vi "Config Data to String.vi"(1 "data":T1[](array[typedef]), 2 "section names":string[](array[string])) -> (0 "string":string)   [LabVIEW 2009]
uses:
  Config Data Section.ctl
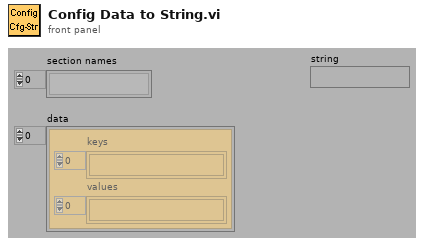
[diagram p1: front panel]
types:
  T1 = typedef "Config Data Section.ctl" = cluster{"keys":string[], "values":string[]}
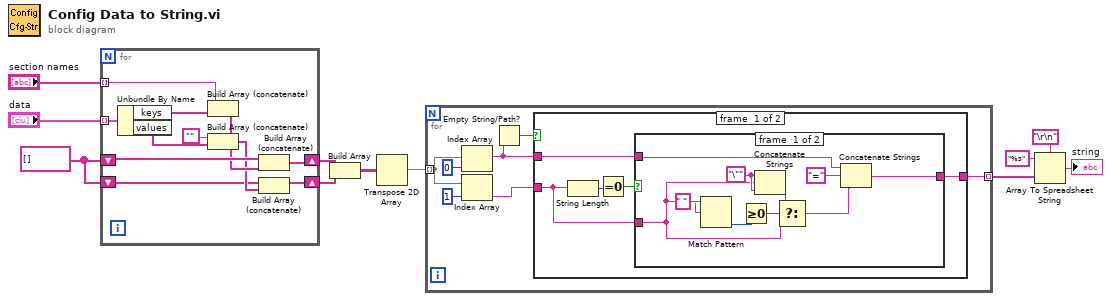
[diagram p0: block diagram]
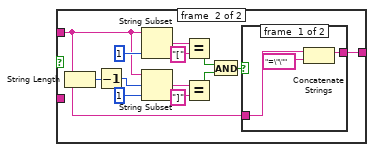
[diagram p2: hidden frame]
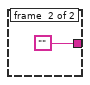
[diagram p4: hidden frame]
diagram:
  w3 = string[] []
  n1 = for {
    tunnel: "data" -> [w22] mode=indexing
    shift-right: [w18] -> w4
    shift-left: w3 -> [w17]
    shift-right: [w13] -> w5
    shift-left: w3 -> [w14]
    tunnel: "section names" -> [w12] mode=indexing
    n2 = Unbundle By Name(w22) -> ("keys"=w21:string[], "values"=w20:string[])
    n3 = Build Array (concatenate)(w12, w21) -> (w16:string[])
    n4 = Build Array (concatenate)("", w20) -> (w15:string[])
    n5 = Build Array (concatenate)(w17, w16) -> (w18:string[])
    n6 = Build Array (concatenate)(w14, w15) -> (w13:string[])
  }
  n7 = Build Array(w4, w5) -> (w6:string[][])
  n8 = Transpose 2D Array(2D array=w6) -> (transposed array=w11:string[][])
  n9 = for {
    tunnel: w11 -> [w26] mode=indexing
    tunnel: [w27] -> w8 mode=indexing
    n10 = Index Array(array=w26, index=0) -> (element=w24:string)
    n11 = Index Array(array=w26, index=1) -> (element=w25:string)
    n12 = Empty String/Path?(string/path=w24) -> (empty?=w23:bool)
    n13 = case shown="False" w23 {
      tunnel: [w32 ""] -> w27
      tunnel: w25 -> [w30 _]
      tunnel: w24 -> [w31 _]
      frame #0 {
        n14 = String Length(string=w30) -> (length=w34:i32)
        n15 = Equal To 0?(x=w34) -> (x = 0?=w33:bool)
        n16 = case shown="True" w33 {
          tunnel: [w42 w45] -> w32
          tunnel: w31 -> [w44 w53]
          tunnel: w30 -> [w38 _]
          frame #0 {
            w39 = "\""
            n17 = Match Pattern(string=w38, regular expression=" ") -> (offset past match=w36:i32)  [unwired: 1 in, 3 out]
            n18 = Greater Or Equal To 0?(x=w36) -> (x >= 0?=w35:bool)
            n19 = Concatenate Strings(w39, w38, w39) -> (w41:string)
            n20 = Select(t=w41, s=w35, f=w38) -> (s? t:f=w40:string)
            n21 = Concatenate Strings(w44, "=", w40) -> (w42:string)
          }
          frame #1 {
            n22 = String Length(string=w53) -> (length=w57:i32)
            n23 = Decrement(x=w57) -> (x-1=w54:i32)
            n24 = String Subset(string=w53, length (rest)=1 ("length (rest)")) -> (substring=w52:string)  [unwired: 1 in]
            n25 = String Subset(string=w53, offset (0)=w54, length (rest)=1 ("length (rest)")) -> (substring=w50:string)
            n26 = Equal?(x=w52, y="[") -> (x = y?=w48:bool)
            n27 = Equal?(x=w50, y="]") -> (x = y?=w47:bool)
            n28 = And(x=w48, y=w47) -> (x .and. y?=w46:bool)
            n29 = case shown="False" w46 {
              tunnel: w53 -> [w59 w61]
              tunnel: [w60 w61] -> w45
              frame #0 {
                n30 = Concatenate Strings(w59, "=\"\"") -> (w60:string)
              }
              frame #1 {
              }
            }
          }
        }
      }
      frame #1 {
      }
    }
  }
  n31 = Array To Spreadsheet String(delimiter (Tab)="\r\n", array=w8, 3:"%s") -> (spreadsheet string=→"string":string)
